vi "transport char run_subvi_2014_05_29_SMU4_JWa.vi"(0 "VISA session":refnum<visa-resource-name>="GPIB0::17::INSTR", 1 "Y2 axis settings":T3={"Y2 axis on/off"=TRUE, "MINIMUM"=-1e-07, "MAXIMUM"=1e-07, "Variable name"="Ig", "LIN or LOG axis"=""} {"MAXIMUM" format="%.2e"; "MINIMUM" format="%.2e"}, 5 "Var1 sweep settings":T5={"start"=0.0, "stop"=-60.0, "step (linear only)"=-1.0, "sweep spacing (linear: 0)"=0, "sweep mode"=FALSE, "compliance (V)"=100.0, "compliance (A)"=0.001} {"compliance (A)" format="%^.2e"; "compliance (V)" format="%.2f"; "sweep spacing (linear: 0)" items=["linear", "log 10", "log 25", "log 50"]; "step (linear only)" format="%.2f"; "stop" format="%.2f"; "start" format="%.2f"}, 7 "Var2 step settings":T4={"compliance (A)"=0.001, "compliance (V)"=100.0, "start"=0.0, "total points"=7, "step"=-10.0} {"step" format="%.2f"; "start" format="%.2f"; "compliance (V)" format="%.2f"; "compliance (A)" format="%^.2e"}, 9 "integration time":u32(slide) scale=0.0..2.0, 11 "Path":path, 13 "Sample Properties:":T2 {"Date Created" format="%<%Y/%m/%d>T"}) -> (6 "graphic display":cluster{"trace":dbl[], "trace":dbl[]}(graph), 8 "Graph Cluster":T1, 15 "error?":errorcluster)   [LabVIEW 2012]
uses:
  <vilib>/Utility/file.llb/Write To Spreadsheet File (DBL).vi
panel:
  in  "Temp (K)":dbl=100.0 format="%^.2e"
  in  "MAXIMUM":ext format="%.2e"
  in  "MINIMUM":ext=-1e-05 format="%_2e"
  out "Gate Current Plot":cluster{"trace":dbl[], "trace":dbl[]}(graph)
  in  "Y1 axis":string="Id"
  in  "wait time parameter":dbl=1.0
  in  "Value (Either V or A) 4":dbl
  in  "Value (Either V or A) 3":dbl
  in  "Value (Either V or A) 2":dbl
  in  "Value (V or A)":dbl
  in  "compliance (A)":dbl=0.001 format="%^.2e"
  in  "compliance (V)":dbl=100.0 format="%^.2e"
  in  "Iname":string="Is"
  in  "Vname":string="Vs"
  in  "Function":u16(ring)=4 items=["disabled", "Var1", "Var2", "Var1'", "Constant"]
  in  "Mode":u16(ring)=4 items=["V", "I", "VPulse", "IPulse", "Common"]
  in  "Iname 4":string="I4"
  in  "Vname 4":string="V4"
  in  "Function 4":u16(ring)=4 items=["disabled", "Var1", "Var2", "Var1'", "Constant"]
  in  "Mode 4":u16(ring) items=["V", "I", "VPulse", "IPulse", "Common"]
  in  "Iname 3":string="Ig"
  in  "Vname 3":string="Vg"
  in  "Function 3":u16(ring)=2 items=["disabled", "Var1", "Var2", "Var1'", "Constant"]
  in  "Mode 3":u16(ring) items=["V", "I", "VPulse", "IPulse", "Common"]
  in  "Iname 2":string="Id"
  in  "Vname 2":string="Vd"
  in  "Function 2":u16(ring)=1 items=["disabled", "Var1", "Var2", "Var1'", "Constant"]
  in  "Mode 2":u16(ring) items=["V", "I", "VPulse", "IPulse", "Common"]
  in  "reset":bool=TRUE
  # "SMU1"
  # "SMU2"
  # "SMU3"
  # "SMU4"
  # "%"
  # "nm"
  # "Device Properties:"
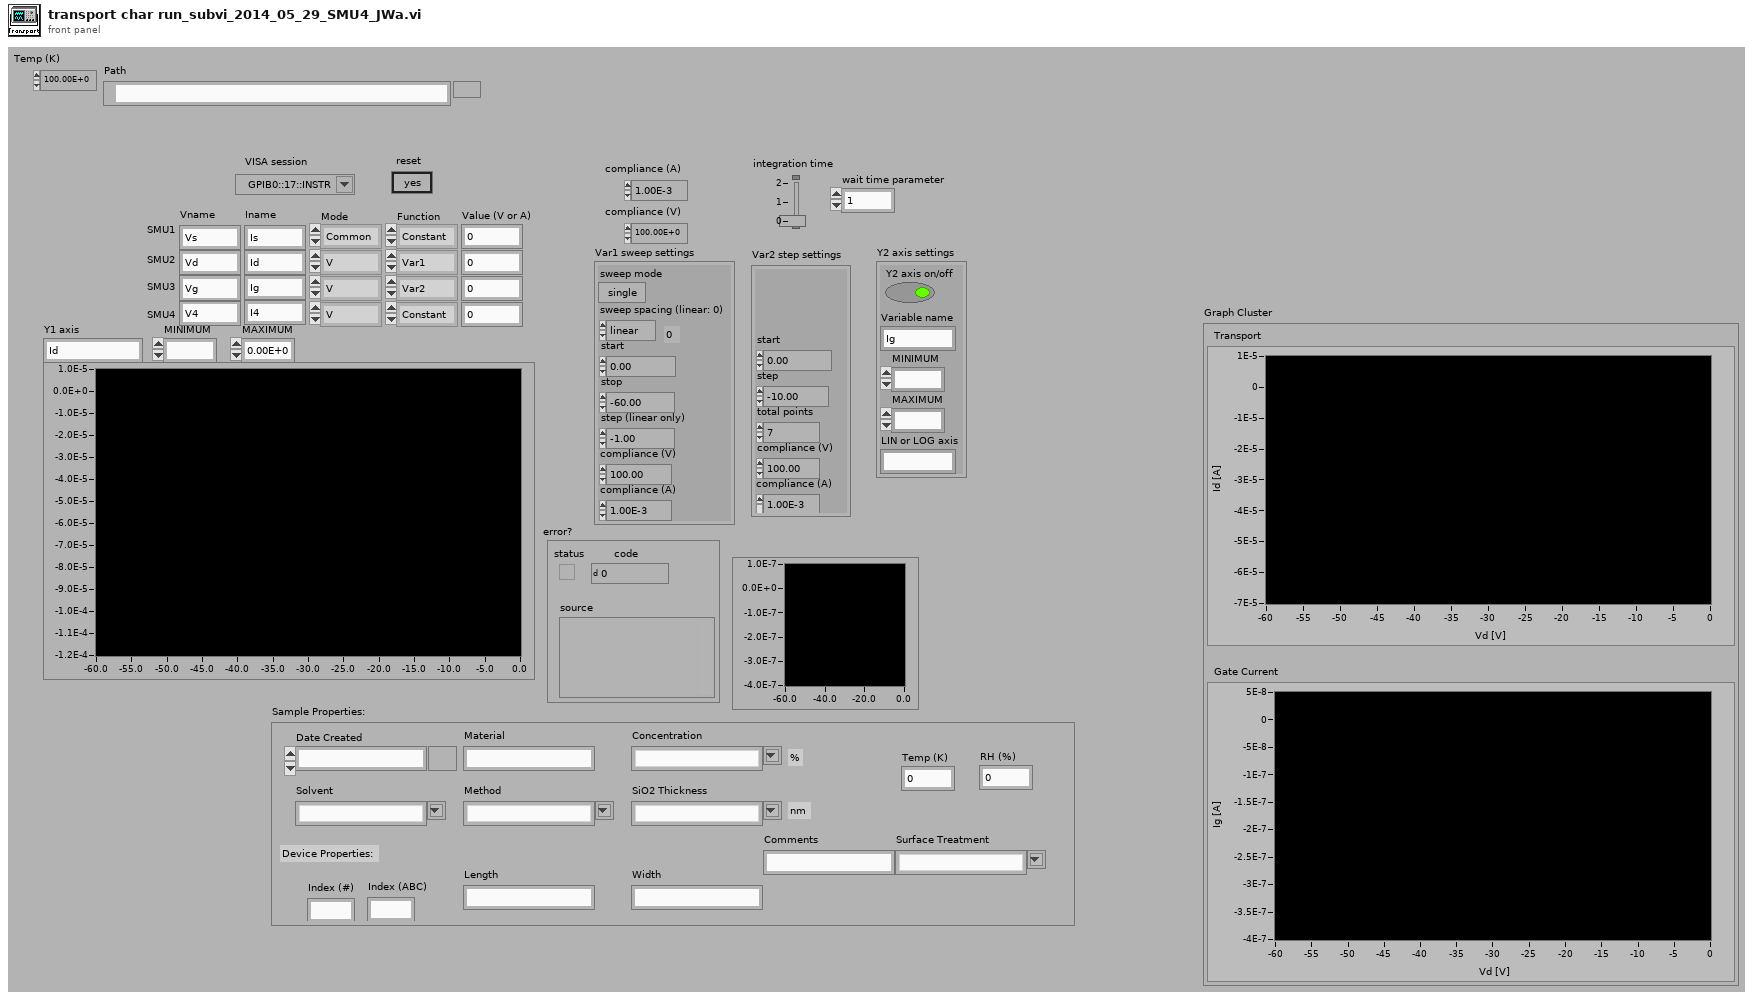
[diagram p1: front panel]
types:
  T1 = cluster{"Transport":cluster{dbl[], dbl[]}[], "Gate Current":cluster{dbl[], dbl[]}[]}
  T2 = cluster{"Date Created":timestamp, "Material":string, "Solvent":string, "Concentration":string, "Method":string, "SiO2 Thickness":string, "Index (#)":string, "Index (ABC)":string, "Length":string, "Width":string, "Surface Treatment":string, "Comments":string, "Temp (K)":dbl, "RH (%)":dbl}
  T3 = cluster{"Y2 axis on/off":bool, "MINIMUM":ext, "MAXIMUM":ext, "Variable name":string, "LIN or LOG axis":string}
  T4 = cluster{"compliance (A)":dbl, "compliance (V)":dbl, "start":dbl, "total points":u16, "step":dbl}
  T5 = cluster{"start":dbl, "stop":dbl, "step (linear only)":dbl, "sweep spacing (linear: 0)":u16, "sweep mode":bool, "compliance (V)":dbl, "compliance (A)":dbl}
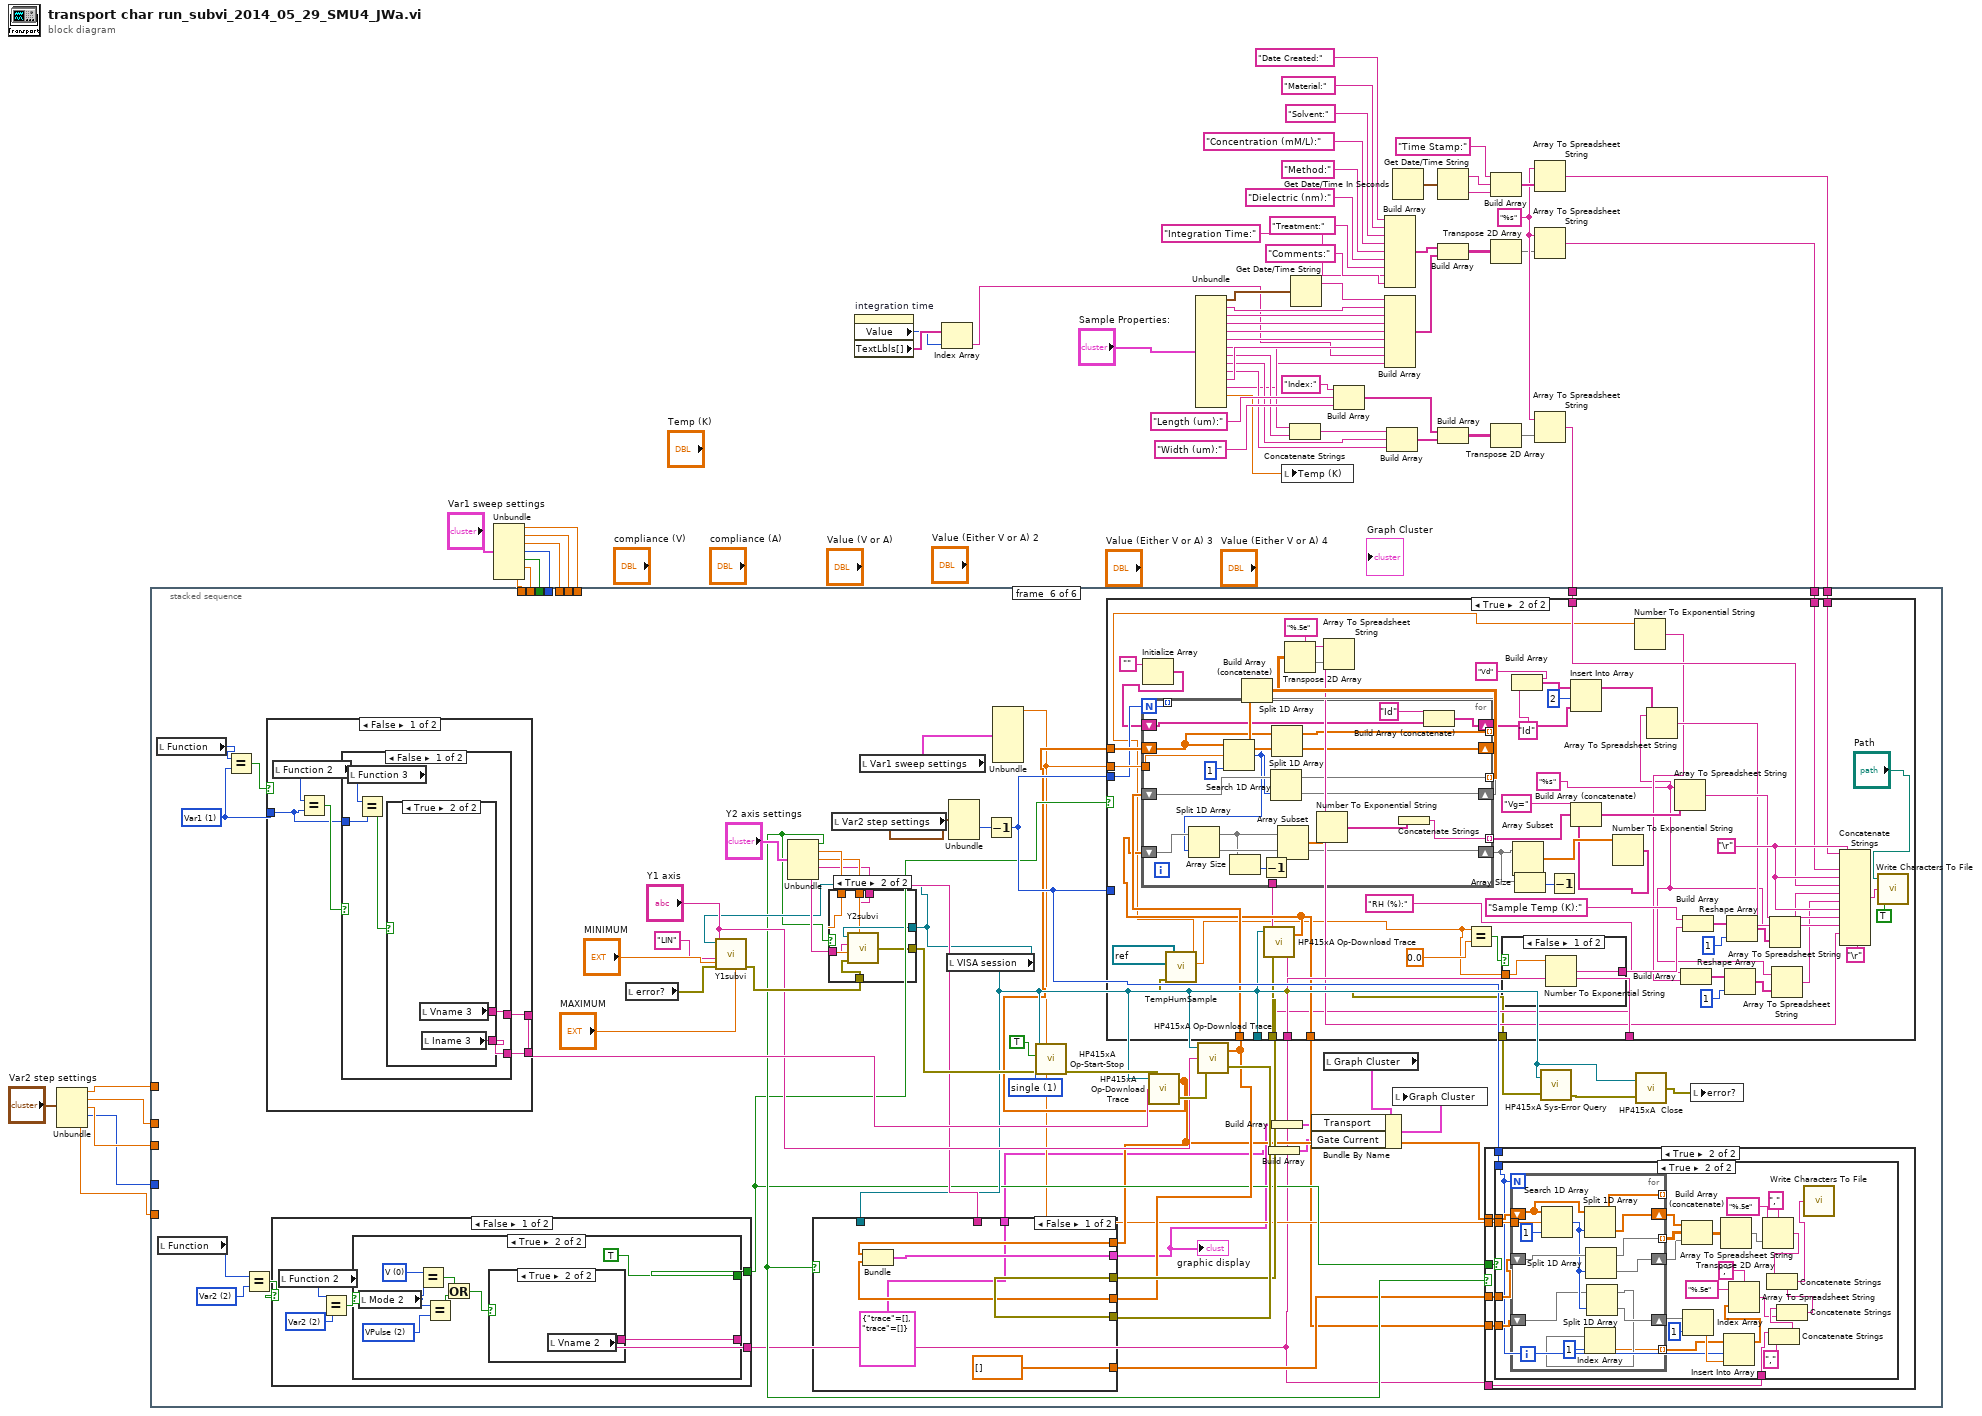
[diagram p0: block diagram]
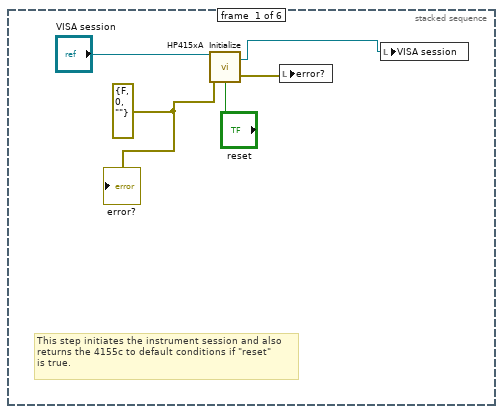
[diagram p2: hidden frame]
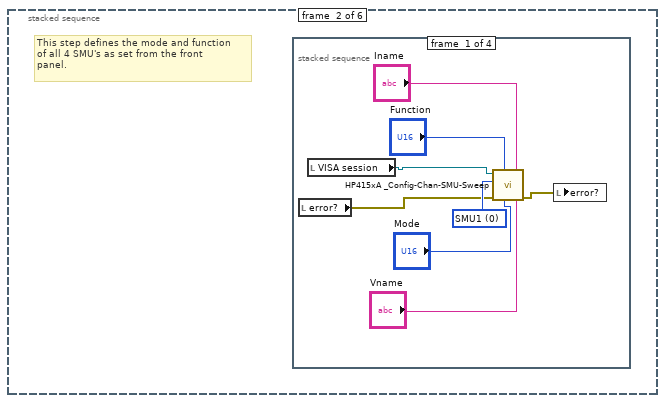
[diagram p3: hidden frame]
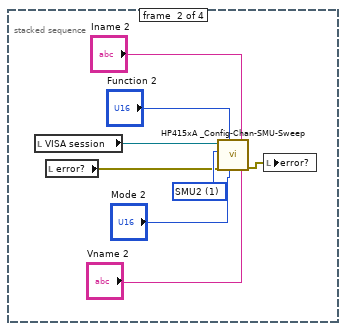
[diagram p4: hidden frame]
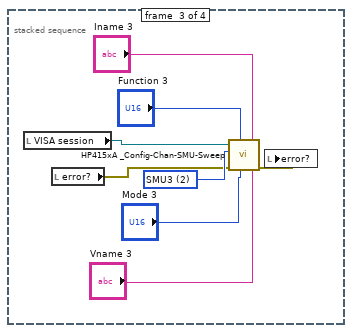
[diagram p5: hidden frame]
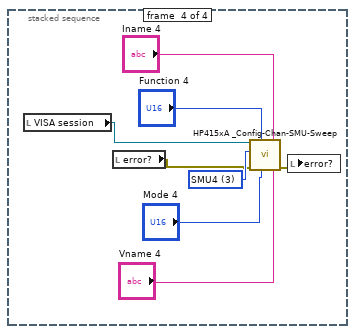
[diagram p6: hidden frame]
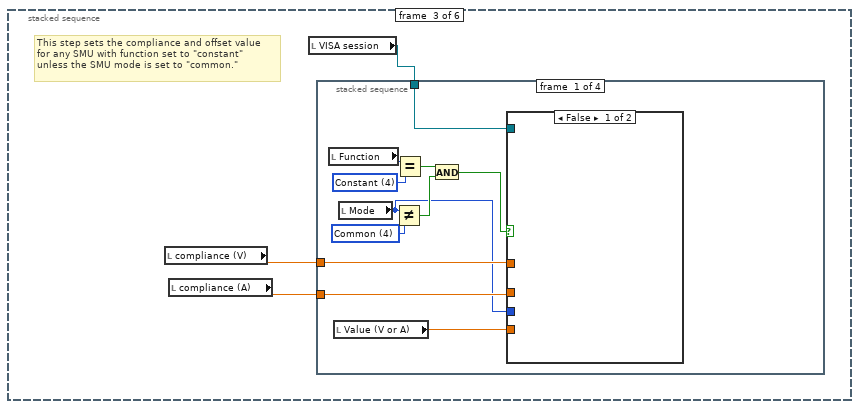
[diagram p7: hidden frame]
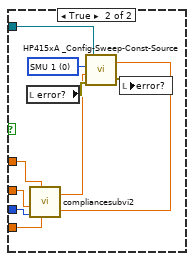
[diagram p8: hidden frame]
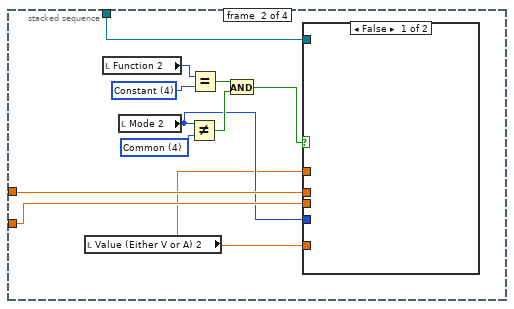
[diagram p9: hidden frame]
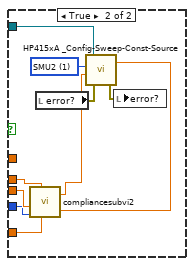
[diagram p10: hidden frame]
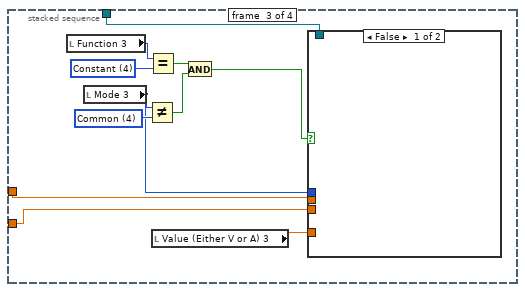
[diagram p11: hidden frame]
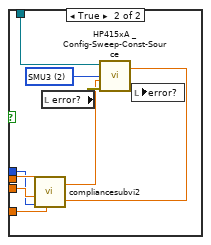
[diagram p12: hidden frame]
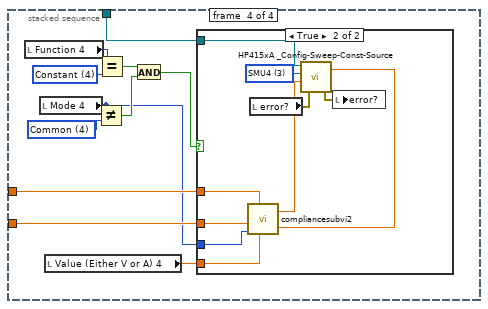
[diagram p13: hidden frame]
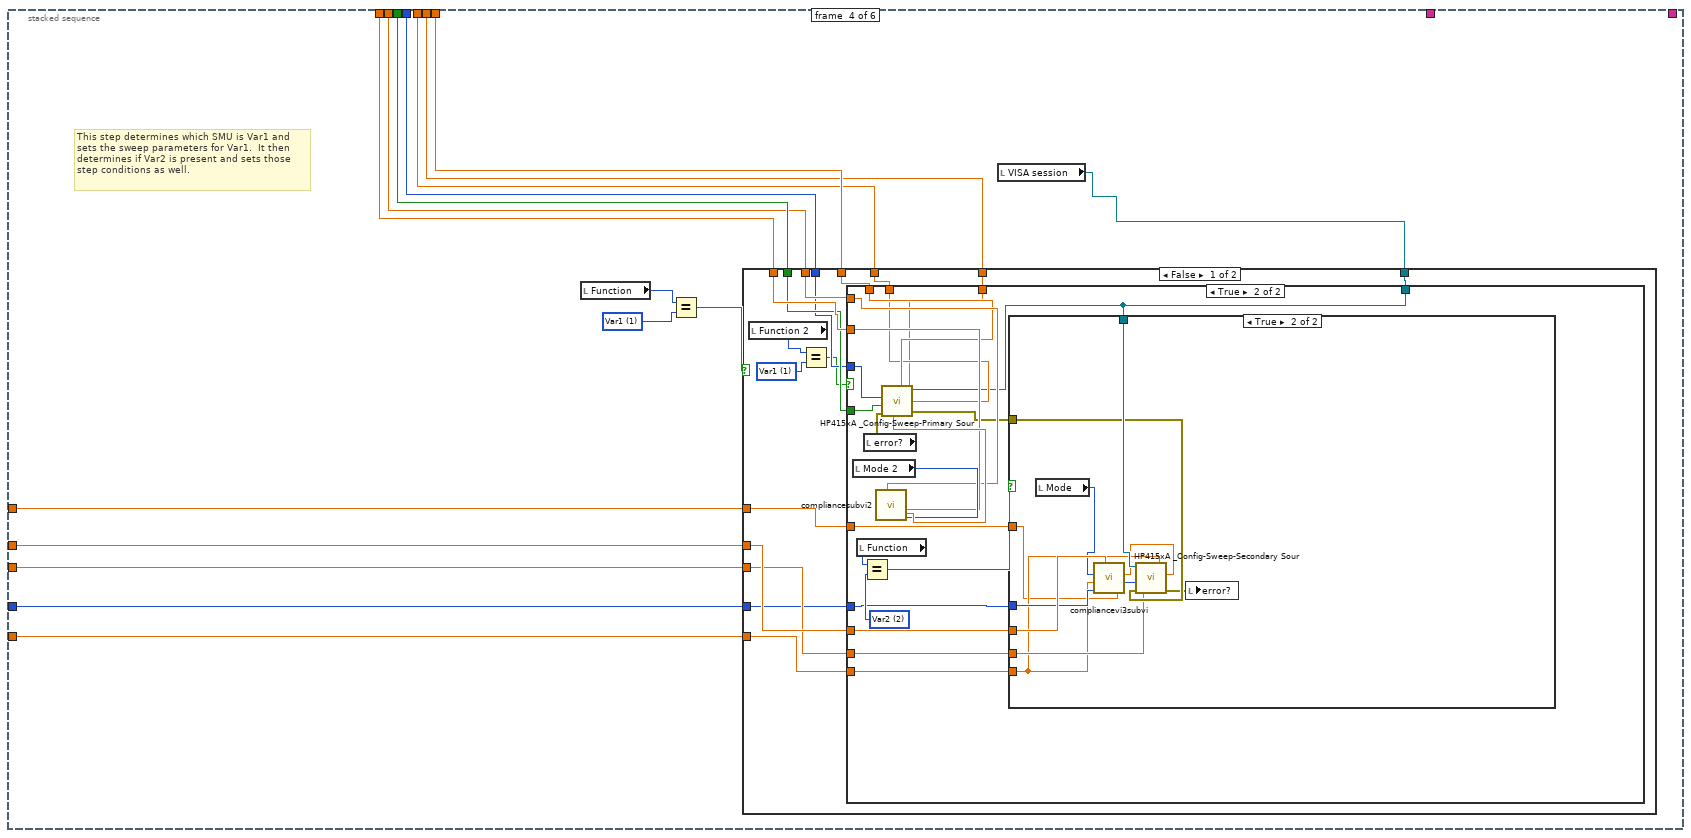
[diagram p15: hidden frame]
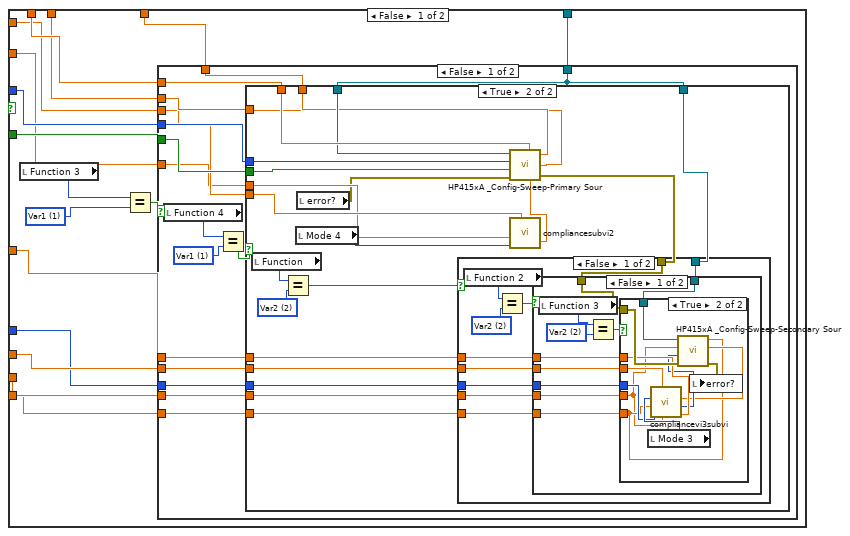
[diagram p16: hidden frame]
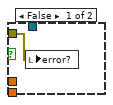
[diagram p18: hidden frame]
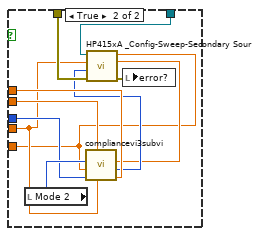
[diagram p19: hidden frame]
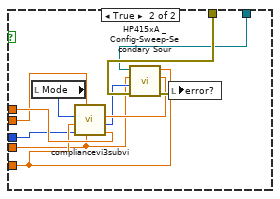
[diagram p20: hidden frame]
diagram:
  w36 = "%s"
  n1 = Unbundle("Var2 step settings") -> ("compliance (A)"=w53:dbl, "compliance (V)"=w52:dbl, "start"=w51:dbl, "total points"=w50:u16, "step"=w49:dbl)
  n2 = Unbundle("Var1 sweep settings") -> ("start"=w61:dbl, "stop"=w60:dbl, "step (linear only)"=w59:dbl, "sweep spacing (linear: 0)"=w58:u16, "sweep mode"=w57:bool, "compliance (V)"=w56:dbl, "compliance (A)"=w55:dbl)
  n3 = property on="integration time" class="Slide (strict)"() -> ("Value"=w4:u32, "TextLbls[]"=w5:string[])  [unwired: 2 in, 2 out]
  n4 = Index Array(array=w5, index=w4) -> (element=w2:string)
  n5 = Unbundle("Sample Properties:") -> ("Date Created"=w20:timestamp, "Material"=w19:string, "Solvent"=w16:string, "Concentration"=w14:string, "Method"=w18:string, "SiO2 Thickness"=w15:string, "Index (#)"=w12:string, "Index (ABC)"=w11:string, "Length"=w9:string, "Width"=w8:string, "Surface Treatment"=w13:string, "Comments"=w3:string, "Temp (K)"=w7:dbl)  [unwired: 1 out]
  n6 = local write "Temp (K)"(w7) -> ()
  n7 = Concatenate Strings(w12, w11) -> (w10:string)
  n8 = Get Date/Time String(seconds (now)=w20) -> (date string=w48:string)  [unwired: 2 in, 1 out]
  n9 = Build Array("Index:", "Length (um):", "Width (um):") -> (w25:string[])
  n10 = Build Array("Date Created:", "Material:", "Solvent:", "Concentration (mM/L):", "Method:", "Dielectric (nm):", "Treatment:", "Integration Time:", "Comments:") -> (w29:string[])
  n11 = Build Array(w48, w19, w16, w14, w18, w15, w13, w2, w3) -> (w28:string[])
  n12 = Build Array(w10, w9, w8) -> (w24:string[])
  n13 = Get Date/Time In Seconds() -> (seconds since 1Jan1904=w43:timestamp)
  n14 = Get Date/Time String(seconds (now)=w43) -> (date string=w42:string, time string=w41:string)  [unwired: 2 in]
  n15 = Build Array(w29, w28) -> (w27:string[][])
  n16 = Build Array(w25, w24) -> (w23:string[][])
  n17 = Build Array("Time Stamp:", w42, w41) -> (w40:string[])
  n18 = Transpose 2D Array(2D array=w27) -> (transposed array=w26:string[][])
  n19 = Transpose 2D Array(2D array=w23) -> (transposed array=w22:string[][])
  n20 = Array To Spreadsheet String(array=w40, 3:w36) -> (spreadsheet string=w35:string)  [unwired: 1 in]
  n21 = Array To Spreadsheet String(array=w26, 3:w36) -> (spreadsheet string=w34:string)  [unwired: 1 in]
  n22 = Array To Spreadsheet String(array=w22, 3:w36) -> (spreadsheet string=w33:string)  [unwired: 1 in]
  n23 = stacked-sequence {
    tunnel: w61 -> [_ _ _ w198 _ _]
    tunnel: w60 -> [_ _ _ w197 _ _]
    tunnel: w59 -> [_ _ _ w196 _ _]
    tunnel: w58 -> [_ _ _ w195 _ _]
    tunnel: w57 -> [_ _ _ w194 _ _]
    tunnel: w56 -> [_ _ _ w193 _ _]
    tunnel: w55 -> [_ _ _ w192 _ _]
    tunnel: w53 -> [_ _ _ w191 _ _]
    tunnel: w52 -> [_ _ _ w190 _ _]
    tunnel: w51 -> [_ _ _ w189 _ _]
    tunnel: w50 -> [_ _ _ w188 _ _]
    tunnel: w49 -> [_ _ _ w187 _ _]
    tunnel: w35 -> [_ _ _ _ _ w561]
    tunnel: w34 -> [_ _ _ _ _ w560]
    tunnel: w33 -> [_ _ _ _ _ w559]
    frame #0 {
      w66 = errorcluster {"status"=FALSE, "code"=0, "source"=""} ("error out")
      # "This step initiates the instrument session and also\nreturns the 4155c to default conditions if \"reset\"\nis true."
      n24 = call "HP415xA  Initialize.vi"("instrument descriptor"="VISA session", "reset"="reset", "error in (no error)"=w66) -> ("VISA session"=w63:refnum<visa-resource-name>, "error out"=w65:errorcluster)  [unwired: 2 in]
      n25 = local write "error?"(w65) -> ()
      n26 = local write "VISA session"(w63) -> ()
      "error?" <- w66
    }
    frame #1 {
      # "This step defines the mode and function\nof all 4 SMU's as set from the front\npanel."
      n27 = stacked-sequence {
        frame #0 {
          w75 = u32 0 items=["SMU1  ", "SMU2  ", "SMU3  ", "SMU4  ", "SMU5  ", "SMU6  "] ("unit to configure")
          n28 = local read "error?"() -> (w70:errorcluster)
          n29 = local read "VISA session"() -> (w68:refnum<visa-resource-name>)
          n30 = call "HP415xA _Config-Chan-SMU-Sweep.vi"("V name (max 6 chars)"="Vname", "I name (max 6 chars)"="Iname", "mode"="Mode", "function"="Function", "error in (no error)"=w70, "unit to configure"=w75, "VISA session"=w68) -> ("error out"=w69:errorcluster)  [unwired: 2 in]
          n31 = local write "error?"(w69) -> ()
        }
        frame #1 {
          w79 = u32 1 items=["SMU1  ", "SMU2  ", "SMU3  ", "SMU4  ", "SMU5  ", "SMU6  "] ("unit to configure")
          n32 = local read "VISA session"() -> (w76:refnum<visa-resource-name>)
          n33 = local read "error?"() -> (w77:errorcluster)
          n34 = call "HP415xA _Config-Chan-SMU-Sweep.vi"("V name (max 6 chars)"="Vname 2", "I name (max 6 chars)"="Iname 2", "mode"="Mode 2", "function"="Function 2", "error in (no error)"=w77, "unit to configure"=w79, "VISA session"=w76) -> ("error out"=w78:errorcluster)  [unwired: 2 in]
          n35 = local write "error?"(w78) -> ()
        }
        frame #2 {
          w87 = u32 2 items=["SMU1  ", "SMU2  ", "SMU3  ", "SMU4  ", "SMU5  ", "SMU6  "] ("unit to configure")
          n36 = local read "VISA session"() -> (w84:refnum<visa-resource-name>)
          n37 = local read "error?"() -> (w85:errorcluster)
          n38 = call "HP415xA _Config-Chan-SMU-Sweep.vi"("V name (max 6 chars)"="Vname 3", "I name (max 6 chars)"="Iname 3", "mode"="Mode 3", "function"="Function 3", "error in (no error)"=w85, "unit to configure"=w87, "VISA session"=w84) -> ("error out"=w86:errorcluster)  [unwired: 2 in]
          n39 = local write "error?"(w86) -> ()
        }
        frame #3 {
          w95 = u32 3 items=["SMU1  ", "SMU2  ", "SMU3  ", "SMU4  ", "SMU5  ", "SMU6  "] ("unit to configure")
          n40 = local read "VISA session"() -> (w92:refnum<visa-resource-name>)
          n41 = local read "error?"() -> (w94:errorcluster)
          n42 = call "HP415xA _Config-Chan-SMU-Sweep.vi"("V name (max 6 chars)"="Vname 4", "I name (max 6 chars)"="Iname 4", "mode"="Mode 4", "function"="Function 4", "error in (no error)"=w94, "unit to configure"=w95, "VISA session"=w92) -> ("error out"=w93:errorcluster)  [unwired: 2 in]
          n43 = local write "error?"(w93) -> ()
        }
      }
    }
    frame #2 {
      # "This step sets the compliance and offset value\nfor any SMU with function set to \"constant\"\nunless the SMU mode is set to \"common.\""
      n44 = local read "compliance (V)"() -> (w101:dbl)
      n45 = local read "compliance (A)"() -> (w102:dbl)
      n46 = local read "VISA session"() -> (w100:refnum<visa-resource-name>)
      n47 = stacked-sequence {
        tunnel: w100 -> [w111 w131 w150 w170]
        tunnel: w102 -> [w105 w127 w148 w168]
        tunnel: w101 -> [w104 w126 w147 w169]
        frame #0 {
          w109 = u16 4 items=["V", "I", "VPulse", "IPulse", "Common"] ("Mode")
          w113 = u16 4 items=["disabled", "Var1", "Var2", "Var1'", "Constant"] ("Function")
          n48 = local read "Function"() -> (w112:u16)
          n49 = local read "Value (V or A)"() -> (w106:dbl)
          n50 = local read "Mode"() -> (w103:u16)
          n51 = Not Equal?(x=w103, y=w109) -> (x != y?=w108:bool)
          n52 = Equal?(x=w112, y=w113) -> (x = y?=w110:bool)
          n53 = And(x=w110, y=w108) -> (x .and. y?=w107:bool)
          n54 = case shown="False" w107 {
            tunnel: w111 -> [_ w123]
            tunnel: w104 -> [_ w119]
            tunnel: w105 -> [_ w118]
            tunnel: w106 -> [_ w115]
            tunnel: w103 -> [_ w116]
            frame False {
            }
            frame True {
              w122 = u16 0 items=["SMU 1", "SMU2", "SMU3", "SMU4", "SMU5", "SMU6", "VSU1", "VSU2"] ("unit (SMU1:0)")
              n55 = local read "error?"() -> (w121:errorcluster)
              n56 = call "compliancesubvi2.vi"("Value1"=w115, "compliance (V)"=w119, "Mode"=w116, "compliance (A)"=w118) -> ("compliance"=w117:dbl, "constant"=w114:dbl)  [unwired: 2 in]
              n57 = call "HP415xA _Config-Sweep-Const-Source.vi"("compliance (SMUs only)"=w117, "error in (no error)"=w121, "source (V or A)"=w114, "unit (SMU1:0)"=w122, "VISA session"=w123) -> ("error out"=w120:errorcluster)
              n58 = local write "error?"(w120) -> ()
            }
          }
        }
        frame #1 {
          w128 = u16 4 items=["V", "I", "VPulse", "IPulse", "Common"] ("Mode 2")
          w129 = u16 4 items=["disabled", "Var1", "Var2", "Var1'", "Constant"] ("Function 2")
          n59 = local read "Value (Either V or A) 2"() -> (w124:dbl)
          n60 = local read "Function 2"() -> (w130:u16)
          n61 = local read "Mode 2"() -> (w125:u16)
          n62 = Not Equal?(x=w125, y=w128) -> (x != y?=w133:bool)
          n63 = Equal?(x=w130, y=w129) -> (x = y?=w134:bool)
          n64 = And(x=w134, y=w133) -> (x .and. y?=w132:bool)
          n65 = case shown="False" w132 {
            tunnel: w131 -> [_ w144]
            tunnel: w126 -> [_ w142]
            tunnel: w127 -> [_ w141]
            tunnel: w124 -> [_ _]
            tunnel: w125 -> [_ w137]
            tunnel: w124 -> [_ w136]
            frame False {
            }
            frame True {
              w143 = u16 1 items=["SMU 1", "SMU2", "SMU3", "SMU4", "SMU5", "SMU6", "VSU1", "VSU2"] ("unit (SMU1:0)")
              n66 = call "compliancesubvi2.vi"("Value1"=w136, "compliance (V)"=w142, "Mode"=w137, "compliance (A)"=w141) -> ("compliance"=w140:dbl, "constant"=w135:dbl)  [unwired: 2 in]
              n67 = local read "error?"() -> (w139:errorcluster)
              n68 = call "HP415xA _Config-Sweep-Const-Source.vi"("compliance (SMUs only)"=w140, "error in (no error)"=w139, "source (V or A)"=w135, "unit (SMU1:0)"=w143, "VISA session"=w144) -> ("error out"=w138:errorcluster)
              n69 = local write "error?"(w138) -> ()
            }
          }
        }
        frame #2 {
          w152 = u16 4 items=["V", "I", "VPulse", "IPulse", "Common"] ("Mode 2")
          w153 = u16 4 items=["disabled", "Var1", "Var2", "Var1'", "Constant"] ("Function 2")
          n70 = local read "Function 3"() -> (w151:u16)
          n71 = local read "Mode 3"() -> (w146:u16)
          n72 = Not Equal?(x=w146, y=w152) -> (x != y?=w154:bool)
          n73 = Equal?(x=w151, y=w153) -> (x = y?=w155:bool)
          n74 = local read "Value (Either V or A) 3"() -> (w149:dbl)
          n75 = And(x=w155, y=w154) -> (x .and. y?=w145:bool)
          n76 = case shown="False" w145 {
            tunnel: w150 -> [_ w163]
            tunnel: w149 -> [_ w157]
            tunnel: w148 -> [_ w160]
            tunnel: w147 -> [_ w159]
            tunnel: w146 -> [_ w158]
            frame False {
            }
            frame True {
              w162 = u16 2 items=["SMU 1", "SMU2", "SMU3", "SMU4", "SMU5", "SMU6", "VSU1", "VSU2"] ("unit (SMU1:0)")
              n77 = call "compliancesubvi2.vi"("Value1"=w157, "compliance (V)"=w159, "Mode"=w158, "compliance (A)"=w160) -> ("compliance"=w161:dbl, "constant"=w156:dbl)  [unwired: 2 in]
              n78 = local read "error?"() -> (w165:errorcluster)
              n79 = call "HP415xA _Config-Sweep-Const-Source.vi"("compliance (SMUs only)"=w161, "error in (no error)"=w165, "source (V or A)"=w156, "unit (SMU1:0)"=w162, "VISA session"=w163) -> ("error out"=w164:errorcluster)
              n80 = local write "error?"(w164) -> ()
            }
          }
        }
        frame #3 {
          w172 = u16 4 items=["V", "I", "VPulse", "IPulse", "Common"] ("Mode 4")
          w173 = u16 4 items=["disabled", "Var1", "Var2", "Var1'", "Constant"] ("Function 4")
          n81 = local read "Function 4"() -> (w174:u16)
          n82 = local read "Mode 4"() -> (w167:u16)
          n83 = local read "Value (Either V or A) 4"() -> (w166:dbl)
          n84 = Not Equal?(x=w167, y=w172) -> (x != y?=w175:bool)
          n85 = Equal?(x=w174, y=w173) -> (x = y?=w176:bool)
          n86 = And(x=w176, y=w175) -> (x .and. y?=w171:bool)
          n87 = case shown="True" w171 {
            tunnel: w170 -> [_ w185]
            tunnel: w169 -> [_ w181]
            tunnel: w168 -> [_ w182]
            tunnel: w167 -> [_ w180]
            tunnel: w166 -> [_ w179]
            frame False {
            }
            frame True {
              w186 = u16 3 items=["SMU 1", "SMU2", "SMU3", "SMU4", "SMU5", "SMU6", "VSU1", "VSU2"] ("unit (SMU1:0)")
              n88 = call "compliancesubvi2.vi"("Value1"=w179, "compliance (V)"=w181, "Mode"=w180, "compliance (A)"=w182) -> ("compliance"=w178:dbl, "constant"=w177:dbl)  [unwired: 2 in]
              n89 = local read "error?"() -> (w184:errorcluster)
              n90 = call "HP415xA _Config-Sweep-Const-Source.vi"("compliance (SMUs only)"=w178, "error in (no error)"=w184, "source (V or A)"=w177, "unit (SMU1:0)"=w186, "VISA session"=w185) -> ("error out"=w183:errorcluster)
              n91 = local write "error?"(w183) -> ()
            }
          }
        }
      }
    }
    frame #3 {
      w202 = u16 1 items=["disabled", "Var1", "Var2", "Var1'", "Constant"] ("Function")
      # "This step determines which SMU is Var1 and\nsets the sweep parameters for Var1.  It then\ndetermines if Var2 is present and sets those\nstep conditions as well."
      n92 = local read "Function"() -> (w201:u16)
      n93 = Equal?(x=w201, y=w202) -> (x = y?=w200:bool)
      n94 = local read "VISA session"() -> (w199:refnum<visa-resource-name>)
      n95 = case shown="False" w200 {
        tunnel: w193 -> [w215 w491]
        tunnel: w192 -> [w216 w490]
        tunnel: w195 -> [w213 w489]
        tunnel: w194 -> [w214 w488]
        tunnel: w196 -> [w210 w487]
        tunnel: w197 -> [w209 w486]
        tunnel: w198 -> [w211 w485]
        tunnel: w199 -> [w212 w474]
        tunnel: w191 -> [w207 w480]
        tunnel: w190 -> [w206 w479]
        tunnel: w189 -> [w205 w478]
        tunnel: w188 -> [w204 w477]
        tunnel: w187 -> [w203 w476]
        frame False {
          w218 = u16 1 items=["disabled", "Var1", "Var2", "Var1'", "Constant"] ("Function")
          n96 = local read "Function 2"() -> (w217:u16)
          n97 = Equal?(x=w217, y=w218) -> (x = y?=w208:bool)
          n98 = case shown="True" w208 {
            tunnel: w216 -> [w224 w417]
            tunnel: w215 -> [w225 w416]
            tunnel: w214 -> [w226 w415]
            tunnel: w213 -> [w227 w414]
            tunnel: w212 -> [w231 w403]
            tunnel: w211 -> [w230 w413]
            tunnel: w210 -> [w228 w412]
            tunnel: w209 -> [w229 w411]
            tunnel: w207 -> [w223 w406]
            tunnel: w206 -> [w222 w405]
            tunnel: w205 -> [w220 w404]
            tunnel: w204 -> [w221 w401]
            tunnel: w203 -> [w219 w400]
            frame False {
              w234 = u16 1 items=["disabled", "Var1", "Var2", "Var1'", "Constant"] ("Function")
              n99 = local read "Function 3"() -> (w233:u16)
              n100 = Equal?(x=w233, y=w234) -> (x = y?=w232:bool)
              n101 = case shown="False" w232 {
                tunnel: w231 -> [w235 w328]
                tunnel: w230 -> [w247 w345]
                tunnel: w229 -> [w244 w344]
                tunnel: w228 -> [w243 w343]
                tunnel: w227 -> [w246 w342]
                tunnel: w226 -> [w245 w341]
                tunnel: w225 -> [w242 w340]
                tunnel: w224 -> [w241 w339]
                tunnel: w223 -> [w240 w332]
                tunnel: w222 -> [w239 w331]
                tunnel: w221 -> [w238 w330]
                tunnel: w220 -> [w237 w327]
                tunnel: w219 -> [w236 w326]
                frame False {
                  w250 = u16 1 items=["disabled", "Var1", "Var2", "Var1'", "Constant"] ("Function")
                  n102 = local read "Function 4"() -> (w249:u16)
                  n103 = Equal?(x=w249, y=w250) -> (x = y?=w248:bool)
                  n104 = case shown="True" w248 {
                    tunnel: w247 -> [_ w269]
                    tunnel: w235 -> [_ w268]
                    tunnel: w246 -> [_ w267]
                    tunnel: w245 -> [_ w266]
                    tunnel: w244 -> [_ w265]
                    tunnel: w243 -> [_ w264]
                    tunnel: w242 -> [_ w263]
                    tunnel: w241 -> [_ w262]
                    tunnel: w240 -> [_ w257]
                    tunnel: w239 -> [_ w256]
                    tunnel: w238 -> [_ w255]
                    tunnel: w237 -> [_ w254]
                    tunnel: w236 -> [_ w253]
                    tunnel: w235 -> [_ w251]
                    frame False {
                    }
                    frame True {
                      w260 = u16 2 items=["disabled", "Var1", "Var2", "Var1'", "Constant"] ("Function")
                      n105 = local read "Function"() -> (w259:u16)
                      n106 = Equal?(x=w259, y=w260) -> (x = y?=w258:bool)
                      n107 = local read "Mode 4"() -> (w271:u16)
                      n108 = local read "error?"() -> (w261:errorcluster)
                      n109 = call "compliancesubvi2.vi"("compliance (V)"=w263, "Mode"=w271, "compliance (A)"=w262) -> ("compliance"=w270:dbl)  [unwired: 3 in, 1 out]
                      n110 = call "HP415xA _Config-Sweep-Primary Sour.vi"("step (linear only)"=w264, "stop"=w265, "start"=w269, "compliance"=w270, "error in (no error)"=w261, "sweep mode"=w266, "sweep spacing (linear: 0)"=w267, "VISA session"=w268) -> ("error out"=w252:errorcluster)  [unwired: 2 in]
                      n111 = case shown="False" w258 {
                        tunnel: w257 -> [w278 w321]
                        tunnel: w256 -> [w277 w316]
                        tunnel: w255 -> [w276 w315]
                        tunnel: w254 -> [w275 w317]
                        tunnel: w253 -> [w274 w320]
                        tunnel: w252 -> [w273 w323]
                        tunnel: w251 -> [w272 w322]
                        frame False {
                          w281 = u16 2 items=["disabled", "Var1", "Var2", "Var1'", "Constant"] ("Function")
                          n112 = local read "Function 2"() -> (w280:u16)
                          n113 = Equal?(x=w280, y=w281) -> (x = y?=w279:bool)
                          n114 = case shown="False" w279 {
                            tunnel: w278 -> [w289 w309]
                            tunnel: w277 -> [w288 w310]
                            tunnel: w276 -> [w287 w308]
                            tunnel: w275 -> [w286 w306]
                            tunnel: w274 -> [w285 w304]
                            tunnel: w273 -> [w284 w314]
                            tunnel: w272 -> [w282 w313]
                            frame False {
                              w291 = u16 2 items=["disabled", "Var1", "Var2", "Var1'", "Constant"] ("Function")
                              n115 = local read "Function 3"() -> (w283:u16)
                              n116 = Equal?(x=w283, y=w291) -> (x = y?=w290:bool)
                              n117 = case shown="True" w290 {
                                tunnel: w289 -> [_ w297]
                                tunnel: w288 -> [_ w298]
                                tunnel: w287 -> [_ w299]
                                tunnel: w286 -> [_ w293]
                                tunnel: w285 -> [_ w294]
                                tunnel: w284 -> [w292 w303]
                                tunnel: w282 -> [_ w302]
                                frame False {
                                n118 = local write "error?"(w292) -> ()
                                }
                                frame True {
                                n119 = local read "Mode 3"() -> (w301:u16)
                                n120 = call "compliancevi3subvi.vi"("compliance (A)"=w297, "start"=w293, "compliance (V)"=w298, "total points"=w299, "step"=w294, "Mode"=w301) -> ("total points 2"=w296:u16, "compliance"=w295:dbl)  [unwired: 1 in, 1 out]
                                n121 = call "HP415xA _Config-Sweep-Secondary Sour.vi"("compliance"=w295, "step"=w294, "error in (no error)"=w303, "total points"=w296, "start"=w293, "VISA session"=w302) -> ("error out"=w300:errorcluster)  [unwired: 1 in]
                                n122 = local write "error?"(w300) -> ()
                                }
                              }
                            }
                            frame True {
                              n123 = local read "Mode 2"() -> (w312:u16)
                              n124 = call "compliancevi3subvi.vi"("compliance (A)"=w309, "start"=w306, "compliance (V)"=w310, "total points"=w308, "step"=w304, "Mode"=w312) -> ("total points 2"=w307:u16, "compliance"=w305:dbl)  [unwired: 1 in, 1 out]
                              n125 = call "HP415xA _Config-Sweep-Secondary Sour.vi"("compliance"=w305, "step"=w304, "error in (no error)"=w314, "total points"=w307, "start"=w306, "VISA session"=w313) -> ("error out"=w311:errorcluster)  [unwired: 1 in]
                              n126 = local write "error?"(w311) -> ()
                            }
                          }
                        }
                        frame True {
                          n127 = local read "Mode"() -> (w325:u16)
                          n128 = call "compliancevi3subvi.vi"("compliance (A)"=w321, "start"=w317, "compliance (V)"=w316, "total points"=w315, "step"=w320, "Mode"=w325) -> ("total points 2"=w318:u16, "compliance"=w319:dbl)  [unwired: 1 in, 1 out]
                          n129 = call "HP415xA _Config-Sweep-Secondary Sour.vi"("compliance"=w319, "step"=w320, "error in (no error)"=w323, "total points"=w318, "start"=w317, "VISA session"=w322) -> ("error out"=w324:errorcluster)  [unwired: 1 in]
                          n130 = local write "error?"(w324) -> ()
                        }
                      }
                    }
                  }
                }
                frame True {
                  w335 = u16 2 items=["disabled", "Var1", "Var2", "Var1'", "Constant"] ("Function")
                  n131 = local read "Function"() -> (w334:u16)
                  n132 = local read "Mode 3"() -> (w337:u16)
                  n133 = call "compliancesubvi2.vi"("compliance (V)"=w340, "Mode"=w337, "compliance (A)"=w339) -> ("compliance"=w338:dbl)  [unwired: 3 in, 1 out]
                  n134 = Equal?(x=w334, y=w335) -> (x = y?=w333:bool)
                  n135 = local read "error?"() -> (w336:errorcluster)
                  n136 = call "HP415xA _Config-Sweep-Primary Sour.vi"("step (linear only)"=w343, "stop"=w344, "start"=w345, "compliance"=w338, "error in (no error)"=w336, "sweep mode"=w341, "sweep spacing (linear: 0)"=w342, "VISA session"=w328) -> ("error out"=w329:errorcluster)  [unwired: 2 in]
                  n137 = case shown="False" w333 {
                    tunnel: w332 -> [w350 w395]
                    tunnel: w331 -> [w349 w394]
                    tunnel: w330 -> [w347 w393]
                    tunnel: w329 -> [w352 w398]
                    tunnel: w328 -> [w351 w397]
                    tunnel: w327 -> [w346 w390]
                    tunnel: w326 -> [w348 w389]
                    frame False {
                      w355 = u16 2 items=["disabled", "Var1", "Var2", "Var1'", "Constant"] ("Function")
                      n138 = local read "Function 2"() -> (w354:u16)
                      n139 = Equal?(x=w354, y=w355) -> (x = y?=w353:bool)
                      n140 = case shown="True" w353 {
                        tunnel: w352 -> [w362 w387]
                        tunnel: w351 -> [w361 w386]
                        tunnel: w350 -> [w360 w382]
                        tunnel: w349 -> [w359 w383]
                        tunnel: w348 -> [w356 w381]
                        tunnel: w347 -> [w358 w384]
                        tunnel: w346 -> [w357 w380]
                        frame False {
                          w365 = u16 2 items=["disabled", "Var1", "Var2", "Var1'", "Constant"] ("Function")
                          n141 = local read "Function 4"() -> (w364:u16)
                          n142 = Equal?(x=w364, y=w365) -> (x = y?=w363:bool)
                          n143 = case shown="True" w363 {
                            tunnel: w362 -> [w366 w375]
                            tunnel: w361 -> [_ w376]
                            tunnel: w360 -> [_ w372]
                            tunnel: w359 -> [_ w373]
                            tunnel: w358 -> [_ w371]
                            tunnel: w357 -> [_ w368]
                            tunnel: w356 -> [_ w367]
                            frame False {
                              n144 = local write "error?"(w366) -> ()
                            }
                            frame True {
                              n145 = local read "Mode 4"() -> (w377:u16)
                              n146 = call "compliancevi3subvi.vi"("compliance (A)"=w372, "start"=w368, "compliance (V)"=w373, "total points"=w371, "step"=w367, "Mode"=w377) -> ("total points 2"=w370:u16, "compliance"=w369:dbl)  [unwired: 1 in, 1 out]
                              n147 = call "HP415xA _Config-Sweep-Secondary Sour.vi"("compliance"=w369, "step"=w367, "error in (no error)"=w375, "total points"=w370, "start"=w368, "VISA session"=w376) -> ("error out"=w374:errorcluster)  [unwired: 1 in]
                              n148 = local write "error?"(w374) -> ()
                            }
                          }
                        }
                        frame True {
                          n149 = local read "Mode 2"() -> (w388:u16)
                          n150 = call "compliancevi3subvi.vi"("compliance (A)"=w382, "start"=w380, "compliance (V)"=w383, "total points"=w384, "step"=w381, "Mode"=w388) -> ("total points 2"=w379:u16, "compliance"=w378:dbl)  [unwired: 1 in, 1 out]
                          n151 = call "HP415xA _Config-Sweep-Secondary Sour.vi"("compliance"=w378, "step"=w381, "error in (no error)"=w387, "total points"=w379, "start"=w380, "VISA session"=w386) -> ("error out"=w385:errorcluster)  [unwired: 1 in]
                          n152 = local write "error?"(w385) -> ()
                        }
                      }
                    }
                    frame True {
                      n153 = local read "Mode"() -> (w399:u16)
                      n154 = call "compliancevi3subvi.vi"("compliance (A)"=w395, "start"=w390, "compliance (V)"=w394, "total points"=w393, "step"=w389, "Mode"=w399) -> ("total points 2"=w392:u16, "compliance"=w391:dbl)  [unwired: 1 in, 1 out]
                      n155 = call "HP415xA _Config-Sweep-Secondary Sour.vi"("compliance"=w391, "step"=w389, "error in (no error)"=w398, "total points"=w392, "start"=w390, "VISA session"=w397) -> ("error out"=w396:errorcluster)  [unwired: 1 in]
                      n156 = local write "error?"(w396) -> ()
                    }
                  }
                }
              }
            }
            frame True {
              w409 = u16 2 items=["disabled", "Var1", "Var2", "Var1'", "Constant"] ("Function")
              n157 = local read "Mode 2"() -> (w418:u16)
              n158 = local read "Function"() -> (w408:u16)
              n159 = Equal?(x=w408, y=w409) -> (x = y?=w407:bool)
              n160 = local read "error?"() -> (w410:errorcluster)
              n161 = call "compliancesubvi2.vi"("compliance (V)"=w416, "Mode"=w418, "compliance (A)"=w417) -> ("compliance"=w419:dbl)  [unwired: 3 in, 1 out]
              n162 = call "HP415xA _Config-Sweep-Primary Sour.vi"("step (linear only)"=w412, "stop"=w411, "start"=w413, "compliance"=w419, "error in (no error)"=w410, "sweep mode"=w415, "sweep spacing (linear: 0)"=w414, "VISA session"=w403) -> ("error out"=w402:errorcluster)  [unwired: 2 in]
              n163 = case shown="True" w407 {
                tunnel: w406 -> [w425 w464]
                tunnel: w405 -> [w424 w469]
                tunnel: w404 -> [w422 w470]
                tunnel: w403 -> [w427 w473]
                tunnel: w402 -> [w421 w472]
                tunnel: w401 -> [w423 w468]
                tunnel: w400 -> [w420 w467]
                frame False {
                  w429 = u16 2 items=["disabled", "Var1", "Var2", "Var1'", "Constant"] ("Function")
                  n164 = local read "Function 3"() -> (w428:u16)
                  n165 = Equal?(x=w428, y=w429) -> (x = y?=w426:bool)
                  n166 = case shown="False" w426 {
                    tunnel: w427 -> [w435 w461]
                    tunnel: w425 -> [w434 w458]
                    tunnel: w424 -> [w432 w456]
                    tunnel: w423 -> [w433 w457]
                    tunnel: w422 -> [w430 w454]
                    tunnel: w421 -> [w436 w460]
                    tunnel: w420 -> [w431 w452]
                    frame False {
                      w439 = u16 2 items=["disabled", "Var1", "Var2", "Var1'", "Constant"] ("Function")
                      n167 = local read "Function 4"() -> (w438:u16)
                      n168 = Equal?(x=w438, y=w439) -> (x = y?=w437:bool)
                      n169 = case shown="True" w437 {
                        tunnel: w436 -> [w440 w451]
                        tunnel: w435 -> [_ w450]
                        tunnel: w434 -> [_ w447]
                        tunnel: w433 -> [_ w448]
                        tunnel: w432 -> [_ w446]
                        tunnel: w431 -> [_ w442]
                        tunnel: w430 -> [_ w443]
                        frame False {
                          n170 = local write "error?"(w440) -> ()
                        }
                        frame True {
                          n171 = local read "Mode 4"() -> (w445:u16)
                          n172 = call "compliancevi3subvi.vi"("compliance (A)"=w447, "start"=w443, "compliance (V)"=w446, "total points"=w448, "step"=w442, "Mode"=w445) -> ("total points 2"=w444:u16, "compliance"=w441:dbl)  [unwired: 1 in, 1 out]
                          n173 = call "HP415xA _Config-Sweep-Secondary Sour.vi"("compliance"=w441, "step"=w442, "error in (no error)"=w451, "total points"=w444, "start"=w443, "VISA session"=w450) -> ("error out"=w449:errorcluster)  [unwired: 1 in]
                          n174 = local write "error?"(w449) -> ()
                        }
                      }
                    }
                    frame True {
                      n175 = local read "Mode 3"() -> (w462:u16)
                      n176 = call "compliancevi3subvi.vi"("compliance (A)"=w458, "start"=w454, "compliance (V)"=w456, "total points"=w457, "step"=w452, "Mode"=w462) -> ("total points 2"=w455:u16, "compliance"=w453:dbl)  [unwired: 1 in, 1 out]
                      n177 = call "HP415xA _Config-Sweep-Secondary Sour.vi"("compliance"=w453, "step"=w452, "error in (no error)"=w460, "total points"=w455, "start"=w454, "VISA session"=w461) -> ("error out"=w459:errorcluster)  [unwired: 1 in]
                      n178 = local write "error?"(w459) -> ()
                    }
                  }
                }
                frame True {
                  n179 = local read "Mode"() -> (w463:u16)
                  n180 = call "compliancevi3subvi.vi"("compliance (A)"=w464, "compliance (V)"=w469, "total points"=w468, "step"=w467, "Mode"=w463) -> ("total points 2"=w465:u16, "compliance"=w466:dbl)  [unwired: 2 in, 1 out]
                  n181 = call "HP415xA _Config-Sweep-Secondary Sour.vi"("compliance"=w466, "step"=w467, "error in (no error)"=w472, "total points"=w465, "start"=w470, "VISA session"=w473) -> ("error out"=w471:errorcluster)  [unwired: 1 in]
                  n182 = local write "error?"(w471) -> ()
                }
              }
            }
          }
        }
        frame True {
          w482 = u16 2 items=["disabled", "Var1", "Var2", "Var1'", "Constant"] ("Function 2")
          n183 = local read "error?"() -> (w484:errorcluster)
          n184 = local read "Mode"() -> (w492:u16)
          n185 = local read "Function 2"() -> (w483:u16)
          n186 = call "compliancesubvi2.vi"("compliance (V)"=w491, "Mode"=w492, "compliance (A)"=w490) -> ("compliance"=w493:dbl)  [unwired: 3 in, 1 out]
          n187 = call "HP415xA _Config-Sweep-Primary Sour.vi"("step (linear only)"=w487, "stop"=w486, "start"=w485, "compliance"=w493, "error in (no error)"=w484, "sweep mode"=w488, "sweep spacing (linear: 0)"=w489, "VISA session"=w474) -> ("error out"=w475:errorcluster)  [unwired: 2 in]
          n188 = Equal?(x=w483, y=w482) -> (x = y?=w481:bool)
          n189 = case shown="True" w481 {
            tunnel: w480 -> [w499 w543]
            tunnel: w479 -> [w500 w542]
            tunnel: w478 -> [w497 w539]
            tunnel: w477 -> [w498 w541]
            tunnel: w476 -> [w496 w537]
            tunnel: w475 -> [w495 w546]
            tunnel: w474 -> [w494 w544]
            frame False {
              w503 = u16 2 items=["disabled", "Var1", "Var2", "Var1'", "Constant"] ("Function 2")
              n190 = local read "Function 3"() -> (w502:u16)
              n191 = Equal?(x=w502, y=w503) -> (x = y?=w501:bool)
              n192 = case shown="True" w501 {
                tunnel: w500 -> [w508 w526]
                tunnel: w499 -> [w509 w527]
                tunnel: w498 -> [w506 w532]
                tunnel: w497 -> [w507 w529]
                tunnel: w496 -> [w505 w528]
                tunnel: w495 -> [w510 w535]
                tunnel: w494 -> [w504 w533]
                frame False {
                  w513 = u16 2 items=["disabled", "Var1", "Var2", "Var1'", "Constant"] ("Function 2")
                  n193 = local read "Function 4"() -> (w512:u16)
                  n194 = Equal?(x=w512, y=w513) -> (x = y?=w511:bool)
                  n195 = case shown="True" w511 {
                    tunnel: w510 -> [w514 w525]
                    tunnel: w509 -> [_ w515]
                    tunnel: w508 -> [_ w516]
                    tunnel: w507 -> [_ w517]
                    tunnel: w506 -> [_ w522]
                    tunnel: w505 -> [_ w519]
                    tunnel: w504 -> [_ w523]
                    frame False {
                      n196 = local write "error?"(w514) -> ()
                    }
                    frame True {
                      n197 = local read "Mode 4"() -> (w521:u16)
                      n198 = call "compliancevi3subvi.vi"("compliance (A)"=w515, "start"=w517, "compliance (V)"=w516, "total points"=w522, "step"=w519, "Mode"=w521) -> ("total points 2"=w518:u16, "compliance"=w520:dbl)  [unwired: 1 in, 1 out]
                      n199 = call "HP415xA _Config-Sweep-Secondary Sour.vi"("compliance"=w520, "step"=w519, "error in (no error)"=w525, "total points"=w518, "start"=w517, "VISA session"=w523) -> ("error out"=w524:errorcluster)  [unwired: 1 in]
                      n200 = local write "error?"(w524) -> ()
                    }
                  }
                }
                frame True {
                  n201 = local read "Mode 3"() -> (w536:u16)
                  n202 = call "compliancevi3subvi.vi"("compliance (A)"=w527, "start"=w529, "compliance (V)"=w526, "total points"=w532, "step"=w528, "Mode"=w536) -> ("total points 2"=w531:u16, "compliance"=w530:dbl)  [unwired: 1 in, 1 out]
                  n203 = call "HP415xA _Config-Sweep-Secondary Sour.vi"("compliance"=w530, "step"=w528, "error in (no error)"=w535, "total points"=w531, "start"=w529, "VISA session"=w533) -> ("error out"=w534:errorcluster)  [unwired: 1 in]
                  n204 = local write "error?"(w534) -> ()
                }
              }
            }
            frame True {
              n205 = local read "Mode 2"() -> (w547:u16)
              n206 = call "compliancevi3subvi.vi"("compliance (A)"=w543, "start"=w539, "compliance (V)"=w542, "total points"=w541, "step"=w537, "Mode"=w547) -> ("total points 2"=w540:u16, "compliance"=w538:dbl)  [unwired: 1 in, 1 out]
              n207 = call "HP415xA _Config-Sweep-Secondary Sour.vi"("compliance"=w538, "step"=w537, "error in (no error)"=w546, "total points"=w540, "start"=w539, "VISA session"=w544) -> ("error out"=w545:errorcluster)  [unwired: 1 in]
              n208 = local write "error?"(w545) -> ()
            }
          }
        }
      }
    }
    frame #4 {
      # "This step sets the integration time."
      n209 = local read "VISA session"() -> (w548:refnum<visa-resource-name>)
      n210 = local read "error?"() -> (w552:errorcluster)
      n211 = call "HP415xA _Config-Meas-Timing.vi"("error in (no error)"=w552, "wait time parameter"="wait time parameter", "integration time"="integration time", "VISA session"=w548) -> ("error out"=w551:errorcluster)  [unwired: 2 in]
      n212 = local write "error?"(w551) -> ()
    }
    frame #5 {
      w588 = u32 1 items=["stop  ", "single  ", "single-append  ", "stress start  ", "continuous  ", "standby on  ", "standby off  ", "zero  "] ("function (stop:0)")
      w592 = u16 2 items=["disabled", "Var1", "Var2", "Var1'", "Constant"] ("Function")
      w597 = u16 1 items=["disabled", "Var1", "Var2", "Var1'", "Constant"] ("Function")
      n213 = local read "Function"() -> (w599:u16)
      n214 = local read "Function"() -> (w591:u16)
      n215 = Equal?(x=w599, y=w597) -> (x = y?=w598:bool)
      n216 = Equal?(x=w591, y=w592) -> (x = y?=w590:bool)
      n217 = case shown="False" w598 {
        tunnel: [w835 w850] -> w593
        tunnel: [w836 w849] -> _
        tunnel: w597 -> [w833 _]
        frame False {
          n218 = local read "Function 2"() -> (w837:u16)
          n219 = Equal?(x=w837, y=w833) -> (x = y?=w834:bool)
          n220 = case shown="False" w834 {
            tunnel: [w838 w848] -> w836
            tunnel: [w839 w847] -> w835
            tunnel: w833 -> [w842 _]
            frame False {
              n221 = local read "Function 3"() -> (w841:u16)
              n222 = Equal?(x=w841, y=w842) -> (x = y?=w840:bool)
              n223 = case shown="True" w840 {
                tunnel: [w844 w846] -> w839
                tunnel: [w843 w845] -> w838
                frame False {
                  n224 = local read "Vname 4"() -> (w844:string)
                  n225 = local read "Iname 4"() -> (w843:string)
                }
                frame True {
                  n226 = local read "Vname 3"() -> (w846:string)
                  n227 = local read "Iname 3"() -> (w845:string)
                }
              }
            }
            frame True {
              n228 = local read "Vname 2"() -> (w847:string)
              n229 = local read "Iname 2"() -> (w848:string)
            }
          }
        }
        frame True {
          n230 = local read "Vname"() -> (w850:string)
          n231 = local read "Iname"() -> (w849:string)
        }
      }
      n232 = case shown="False" w590 {
        tunnel: [w685 w738] -> w564
        tunnel: [w684 TRUE ("x = y?")] -> w569
        frame False {
          w688 = u16 2 items=["disabled", "Var1", "Var2", "Var1'", "Constant"] ("Function")
          n233 = local read "Function 2"() -> (w687:u16)
          n234 = Equal?(x=w687, y=w688) -> (x = y?=w686:bool)
          n235 = case shown="True" w686 {
            tunnel: [w690 w728] -> w685
            tunnel: [w689 TRUE ("x = y?")] -> w684
            frame False {
              w693 = u16 2 items=["disabled", "Var1", "Var2", "Var1'", "Constant"] ("Function")
              n236 = local read "Function 3"() -> (w692:u16)
              n237 = Equal?(x=w692, y=w693) -> (x = y?=w691:bool)
              n238 = case shown="False" w691 {
                tunnel: [w698 w718] -> w690
                tunnel: [w694 TRUE ("x = y?")] -> w689
                frame False {
                  w697 = u16 2 items=["disabled", "Var1", "Var2", "Var1'", "Constant"] ("Function")
                  n239 = local read "Function 4"() -> (w696:u16)
                  n240 = Equal?(x=w696, y=w697) -> (x = y?=w695:bool)
                  n241 = case shown="True" w695 {
                    tunnel: ["0" ("Vname 4") w708] -> w698
                    tunnel: [FALSE ("x = y?") TRUE ("x = y?")] -> w694
                    frame False {
                    }
                    frame True {
                      w702 = u16 2 items=["V", "I", "VPulse", "IPulse", "Common"] ("Mode 2")
                      w705 = u16 0 items=["V", "I", "VPulse", "IPulse", "Common"] ("Mode 2")
                      n242 = local read "Mode 4"() -> (w704:u16)
                      n243 = Equal?(x=w705, y=w704) -> (x = y?=w706:bool)
                      n244 = Equal?(x=w704, y=w702) -> (x = y?=w703:bool)
                      n245 = Or(x=w706, y=w703) -> (x .or. y?=w701:bool)
                      n246 = case shown="False" w701 {
                        tunnel: [w709 w710] -> w708
                        frame False {
                          n247 = local read "Iname 4"() -> (w709:string)
                        }
                        frame True {
                          n248 = local read "Vname 4"() -> (w710:string)
                        }
                      }
                    }
                  }
                }
                frame True {
                  w714 = u16 2 items=["V", "I", "VPulse", "IPulse", "Common"] ("Mode 2")
                  w713 = u16 0 items=["V", "I", "VPulse", "IPulse", "Common"] ("Mode 2")
                  n249 = local read "Mode 3"() -> (w712:u16)
                  n250 = Equal?(x=w713, y=w712) -> (x = y?=w716:bool)
                  n251 = Equal?(x=w712, y=w714) -> (x = y?=w715:bool)
                  n252 = Or(x=w716, y=w715) -> (x .or. y?=w711:bool)
                  n253 = case shown="False" w711 {
                    tunnel: [w719 w720] -> w718
                    frame False {
                      n254 = local read "Iname 3"() -> (w719:string)
                    }
                    frame True {
                      n255 = local read "Vname 3"() -> (w720:string)
                    }
                  }
                }
              }
            }
            frame True {
              w722 = u16 2 items=["V", "I", "VPulse", "IPulse", "Common"] ("Mode 2")
              w723 = u16 0 items=["V", "I", "VPulse", "IPulse", "Common"] ("Mode 2")
              n256 = local read "Mode 2"() -> (w724:u16)
              n257 = Equal?(x=w723, y=w724) -> (x = y?=w726:bool)
              n258 = Equal?(x=w724, y=w722) -> (x = y?=w725:bool)
              n259 = Or(x=w726, y=w725) -> (x .or. y?=w721:bool)
              n260 = case shown="True" w721 {
                tunnel: [w729 w730] -> w728
                frame False {
                  n261 = local read "Iname 2"() -> (w729:string)
                }
                frame True {
                  n262 = local read "Vname 2"() -> (w730:string)
                }
              }
            }
          }
        }
        frame True {
          w735 = u16 2 items=["V", "I", "VPulse", "IPulse", "Common"] ("Mode")
          w736 = u16 0 items=["V", "I", "VPulse", "IPulse", "Common"] ("Mode")
          n263 = local read "Mode"() -> (w734:u16)
          n264 = Equal?(x=w734, y=w736) -> (x = y?=w733:bool)
          n265 = Equal?(x=w734, y=w735) -> (x = y?=w732:bool)
          n266 = Or(x=w733, y=w732) -> (x .or. y?=w731:bool)
          n267 = case shown="True" w731 {
            tunnel: [w739 w740] -> w738
            frame False {
              n268 = local read "Iname"() -> (w739:string)
            }
            frame True {
              n269 = local read "Vname"() -> (w740:string)
            }
          }
        }
      }
      n270 = local read "error?"() -> (w580:errorcluster)
      n271 = Unbundle("Y2 axis settings") -> ("Y2 axis on/off"=w571:bool, "MINIMUM"=w585:ext, "MAXIMUM"=w584:ext, "Variable name"=w577:string, "LIN or LOG axis"=w583:string)
      n272 = local read "Var2 step settings"() -> (w595:T4)
      n273 = local read "Var1 sweep settings"() -> (w596:T5)
      n274 = local read "VISA session"() -> (w575:refnum<visa-resource-name>)
      n275 = call "Y1subvi.vi"("MAXIMUM"="MAXIMUM", "MINIMUM"="MINIMUM", "error in (no error)"=w580, "LIN or LOG axis"="LIN", "Variable name"="Y1 axis", "VISA In"=w575) -> ("error out"=w581:errorcluster)  [unwired: 4 in, 1 out]
      n276 = case shown="True" w571 {
        tunnel: w581 -> [w676 w683]
        tunnel: w575 -> [_ w682]
        tunnel: w585 -> [_ w681]
        tunnel: w584 -> [_ w680]
        tunnel: w577 -> [_ w679]
        tunnel: w583 -> [_ w678]
        tunnel: [w676 w677] -> w582
        frame False {
        }
        frame True {
          n277 = call "Y2subvi.vi"("MAXIMUM"=w680, "Variable name"=w679, "error in (no error)"=w683, "MINIMUM"=w681, "LIN or LOG axis"=w678, "VISA resource name"=w682) -> ("error out"=w677:errorcluster)
        }
      }
      n278 = Unbundle(w595) -> ("total points"=w594:u16)  [unwired: 4 out]
      n279 = Decrement(x=w594) -> (x-1=w570:u16)
      n280 = Unbundle(w596) -> ("start"=w567:dbl)  [unwired: 6 out]
      n281 = call "HP415xA Op-Start-Stop.vi"("error in (no error)"=w582, "function (stop:0)"=w588, "wait until finish"=TRUE, "VISA session"=w575) -> ("error out"=w587:errorcluster)  [unwired: 6 in, 1 out]
      n282 = call "HP415xA Op-Download Trace.vi"("error in (no error)"=w587, "trace (variable) name"=w593, "VISA session"=w575) -> ("error out"=w602:errorcluster, "trace"=w568:dbl[])
      n283 = call "HP415xA Op-Download Trace.vi"("error in (no error)"=w602, "trace (variable) name"="Y1 axis", "VISA session"=w575) -> ("error out"=w578:errorcluster, "trace"=w572:dbl[])
      n284 = case shown="False" w571 {
        tunnel: w578 -> [w660 w669]
        tunnel: w575 -> [_ w668]
        tunnel: w577 -> [_ w667]
        tunnel: [w660 w666] -> w576
        tunnel: w568 -> [w658 w665]
        tunnel: w572 -> [w659 w664]
        tunnel: [w657 w663] -> w555
        tunnel: [dbl[] [] ("trace") w662] -> w566
        tunnel: [cluster{"trace":dbl[], "trace":dbl[]} {"trace"=[], "trace"=[]} w661] -> w553
        frame False {
          n285 = Bundle("trace"=w658, "trace"=w659) -> (w657:cluster{"trace":dbl[], "trace":dbl[]})  [unwired: 1 in]
        }
        frame True {
          n286 = call "HP415xA Op-Download Trace.vi"("error in (no error)"=w669, "trace (variable) name"=w667, "VISA session"=w668) -> ("error out"=w666:errorcluster, "trace"=w662:dbl[])
          n287 = stacked-sequence {
            tunnel: w662 -> [_ w675]
            tunnel: w665 -> [w672 w674]
            tunnel: w664 -> [w671 _]
            tunnel: [w670 _] -> w663
            tunnel: [_ w673] -> w661
            frame #0 {
              n288 = Bundle("trace"=w672, "trace"=w671) -> (w670:cluster{"trace":dbl[], "trace":dbl[]})  [unwired: 1 in]
            }
            frame #1 {
              n289 = Bundle("trace"=w674, "trace"=w675) -> (w673:cluster{"trace":dbl[], "trace":dbl[]})  [unwired: 1 in]
              "Gate Current Plot" <- w673
            }
          }
        }
      }
      "graphic display" <- w555
      n290 = case shown="True" w569 {
        tunnel: w567 -> [_ w808]
        tunnel: w572 -> [w745 w807]
        tunnel: w568 -> [w746 w805]
        tunnel: w570 -> [_ w803]
        tunnel: w570 -> [_ _]
        tunnel: w575 -> [_ w799]
        tunnel: w576 -> [_ w798]
        tunnel: [w747 w751] -> w563
        tunnel: w564 -> [_ w797]
        tunnel: w564 -> [_ w787]
        tunnel: [dbl[] [] ("trace") w796] -> w565
        tunnel: w561 -> [_ w791]
        tunnel: w560 -> [_ w790]
        tunnel: w559 -> [_ w789]
        frame False {
          n291 = Build Array(w746, w745) -> (w742:dbl[][])
          n292 = local read "error?"() -> (w747:errorcluster)
          n293 = call-poly <vilib>:"Write To Spreadsheet File.vi"("transpose? (no:F)"=TRUE ("append to file? (new file:F)"), "format (%.3f)"="%.5e", "2D data"=w742) -> ()  [unwired: 5 in, 1 out]
        }
        frame True {
          w752 = "%s"
          w793 = "\r"
          n294 = Initialize Array("") -> (w770:string[])  [unwired: 1 in]
          n295 = call "HP415xA Op-Download Trace.vi"("error in (no error)"=w798, "trace (variable) name"=w797, "VISA session"=w799) -> ("error out"=w751:errorcluster, "trace"=w796:dbl[])
          n296 = for {
            N: w803 -> [w812]
            shift-right: [w829] -> w776
            shift-left: w805 -> [w825]
            tunnel: w808 -> [w831]
            tunnel: [w830] -> _ mode=indexing
            shift-right: [w826] -> w804
            shift-left: w807 -> [w828]
            tunnel: [w827] -> w806 mode=indexing
            shift-right: [w822] -> w783
            shift-left: w796 -> [w824]
            tunnel: w787 -> [_]
            tunnel: [w816] -> w785 mode=indexing
            shift-right: [w815] -> w774
            shift-left: w770 -> [w814]
            tunnel: [w812] -> _ mode=indexing
            n297 = Search 1D Array(1D array=w825, element=w831, start index (0)=1) -> (index of element=w823:i32)
            n298 = Split 1D Array(array=w824, index=w823) -> (first subarray=w820:dbl[], second subarray=w822:dbl[])
            n299 = Array Size(array=w820) -> (size(s)=w819:i32)
            n300 = Decrement(x=w819) -> (x-1=w818:i32)
            n301 = Split 1D Array(array=w828, index=w823) -> (first subarray=w827:dbl[], second subarray=w826:dbl[])
            n302 = Split 1D Array(array=w825, index=w823) -> (first subarray=w830:dbl[], second subarray=w829:dbl[])
            n303 = Array Subset(array=w820, index=w818) -> (w821:dbl[])  [unwired: 1 in]
            n304 = Number To Exponential String(number=w821) -> (E-format string=w817:string[])  [unwired: 3 in]
            n305 = Concatenate Strings(w817) -> (w816:string)
            n306 = Build Array (concatenate)("Id", w814) -> (w815:string[])
          }
          n307 = call "TempHumSample.vi"("VISA resource name"=refnum<visa-resource-name> "COM4", "error in (no error)"=w751) -> ("CurHum"=w748:dbl, "CurTemp"=w749:dbl)  [unwired: 6 in, 1 out]
          n308 = Build Array (concatenate)(w776, w806, w804) -> (w802:dbl[][])
          n309 = Transpose 2D Array(2D array=w802) -> (transposed array=w800:dbl[][])
          n310 = Array To Spreadsheet String(array=w800, 3:"%.5e" ("format string")) -> (spreadsheet string=w788:string)  [unwired: 1 in]
          n311 = Equal?(x=w749, y=0.0) -> (x = y?=w762:bool)
          n312 = case shown="False" w762 {
            tunnel: w749 -> [w810 _]
            tunnel: [w809 ""] -> w760
            frame False {
              n313 = Number To Exponential String(number=w810) -> (E-format string=w809:string)  [unwired: 3 in]
            }
            frame True {
            }
          }
          n314 = Build Array("Vd", "Id") -> (w775:string[])
          n315 = Array Size(array=w783) -> (size(s)=w784:i32)
          n316 = Decrement(x=w784) -> (x-1=w782:i32)
          n317 = Array Subset(array=w783, index=w782) -> (w781:dbl[])  [unwired: 1 in]
          n318 = Insert Into Array(array=w775, index=2, new element=w774) -> (w773:string[])
          n319 = Number To Exponential String(number=w781) -> (E-format string=w767:string[])  [unwired: 3 in]
          n320 = Build Array (concatenate)("Vg=", w785, w767) -> (w780:string[])
          n321 = Number To Exponential String(number=w748) -> (E-format string=w753:string)  [unwired: 3 in]
          n322 = Array To Spreadsheet String(array=w773, 3:w752) -> (spreadsheet string=w779:string)  [unwired: 1 in]
          n323 = Array To Spreadsheet String(array=w780, 3:w752) -> (spreadsheet string=w786:string)  [unwired: 1 in]
          n324 = Build Array("RH (%):", w753) -> (w758:string[])
          n325 = Build Array("Sample Temp (K):", w760) -> (w765:string[])
          n326 = Reshape Array(w758, 1 ("start index (0)")) -> (w755:string[])
          n327 = Reshape Array(w765, 1 ("start index (0)")) -> (w763:string[])
          n328 = Array To Spreadsheet String(array=w763, 3:w752) -> (spreadsheet string=w757:string)  [unwired: 1 in]
          n329 = Array To Spreadsheet String(array=w755, 3:w752) -> (spreadsheet string=w756:string)  [unwired: 1 in]
          n330 = Concatenate Strings(w791, w793, w790, w793, w789, w757, w756, w793, w786, w779, w788, "\r") -> (w795:string)
          n331 = call <vilib>:"Write Characters To File.vi"("append to file? (new file:F)"=TRUE, "character string"=w795, "file path (dialog if empty)"="Path") -> ()  [unwired: 2 in, 1 out]
        }
      }
      n332 = Build Array(w553) -> (w554:cluster{"trace":dbl[], "trace":dbl[]}[])
      n333 = Build Array(w555) -> (w556:cluster{"trace":dbl[], "trace":dbl[]}[])
      n334 = local read "Graph Cluster"() -> (w558:T1)
      n335 = Bundle By Name(cluster=w558, "Transport"=w556, "Gate Current"=w554) -> (w557:T1)
      n336 = local write "Graph Cluster"(w557) -> ()
      n337 = case shown="True" w571 {
        tunnel: w570 -> [_ w608]
        tunnel: w569 -> [_ w609]
        tunnel: w568 -> [_ w607]
        tunnel: w567 -> [_ w606]
        tunnel: w566 -> [_ w605]
        tunnel: w565 -> [_ w604]
        tunnel: w564 -> [_ w603]
        frame False {
        }
        frame True {
          n338 = case shown="True" w609 {
            tunnel: w608 -> [_ w625]
            tunnel: w607 -> [w613 w640]
            tunnel: w606 -> [_ w639]
            tunnel: w605 -> [w614 w638]
            tunnel: w604 -> [_ w637]
            tunnel: w603 -> [_ w620]
            frame False {
              n339 = Build Array(w613, w614) -> (w612:dbl[][])
              n340 = call-poly <vilib>:"Write To Spreadsheet File.vi"("transpose? (no:F)"=TRUE, "format (%.3f)"="%.5e", "2D data"=w612) -> ()  [unwired: 5 in, 1 out]
            }
            frame True {
              n341 = for {
                N: w625 -> [_]
                shift-right: [w651] -> w636
                shift-left: w640 -> [w652]
                tunnel: w639 -> [w654]
                tunnel: [w650] -> _ mode=indexing
                shift-right: [w647] -> w634
                shift-left: w638 -> [w649]
                tunnel: [w648] -> w635 mode=indexing
                shift-right: [w644] -> w629
                shift-left: w637 -> [w645]
                tunnel: [w641] -> w626 mode=indexing
                n342 = Search 1D Array(1D array=w652, element=w654, start index (0)=1) -> (index of element=w646:i32)
                n343 = Split 1D Array(array=w652, index=w646) -> (first subarray=w650:dbl[], second subarray=w651:dbl[])
                n344 = Split 1D Array(array=w649, index=w646) -> (first subarray=w648:dbl[], second subarray=w647:dbl[])
                n345 = Split 1D Array(array=w645, index=w646) -> (first subarray=w642:dbl[], second subarray=w644:dbl[])
                n346 = Index Array(array=w642, index=1) -> (element=w641:dbl)
              }
              n347 = Build Array (concatenate)(w636, w635, w634) -> (w633:dbl[][])
              n348 = Index Array(array=w629, index=1) -> (element=w627:dbl)
              n349 = Transpose 2D Array(2D array=w633) -> (transposed array=w632:dbl[][])
              n350 = Insert Into Array(array=w626, index=w625, new element=w627) -> (w624:dbl[])
              n351 = Array To Spreadsheet String(delimiter (Tab)=",", array=w624, 3:"%.5e" ("format string")) -> (spreadsheet string=w618:string)
              n352 = Array To Spreadsheet String(delimiter (Tab)=",", array=w632, 3:"%.5e" ("format string")) -> (spreadsheet string=w616:string)
              n353 = Concatenate Strings(w620, "," ("string")) -> (w619:string)
              n354 = Concatenate Strings(w619, w618) -> (w617:string)
              n355 = Concatenate Strings(w617, w616) -> (w615:string)
              n356 = call <vilib>:"Write Characters To File.vi"("character string"=w615) -> ()  [unwired: 4 in, 1 out]
            }
          }
        }
      }
      n357 = call "HP415xA Sys-Error Query.vi"("VISA session"=w575, "error in (no error)"=w563) -> ("error out"=w600:errorcluster)  [unwired: 2 in, 1 out]
      n358 = call "HP415xA  Close.vi"("error in (no error)"=w600, "VISA session"=w575) -> ("error out"=w601:errorcluster)
      n359 = local write "error?"(w601) -> ()
    }
  }
